vi "GetCaseTerm.vi"(8 "error in (no error)":errorcluster, 9 "CaseStructureName":string, 10 "WireLabel":string, 11 "VI Ref":refnum<vi>) -> (0 "error out":errorcluster, 1 "Open Refs":refnum<vi>[](array[refnum]), 2 "Found?":bool, 3 "Terminal Ref":refnum<vi>)   [LabVIEW 2016, in "CS++Actor.lvlib" / "CS++Actor.lvclass"]
uses:
  CS++Actor.lvclass
  <vilib>/Utility/traverseref.llb/TRef TravTarget.ctl
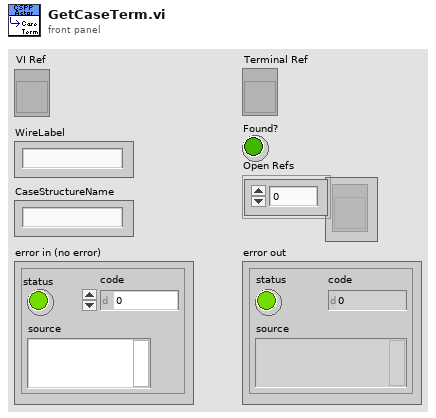
[diagram p1: front panel]
types:
  T1 = typedef "TRef TravTarget.ctl" = enum16{"FP", "BD", "Other"}
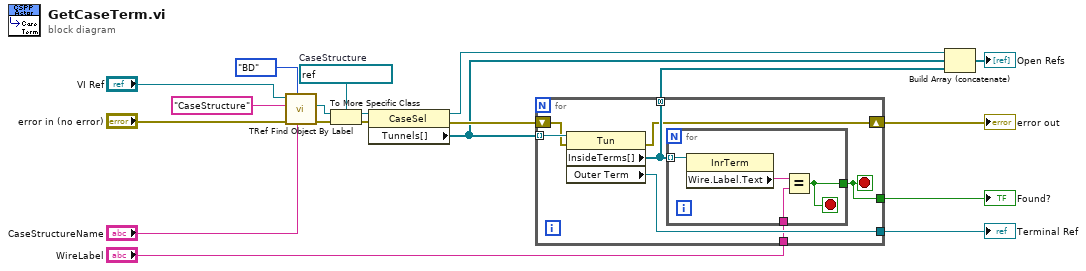
[diagram p0: block diagram]
diagram:
  w17 = refnum<vi> refnum  # CaseStructure
  n1 = call <vilib>:"TRef Find Object By Label.vi"("Label"="CaseStructureName", "Traverse Target"=TRef_TravTarget."BD", "error in (no error)"="error in (no error)", "Class Name"="CaseStructure", "VI Ref"="VI Ref") -> ("error out"=w15:errorcluster, "Found Obj Ref"=w16:refnum<vi>)  [unwired: 3 in, 2 out]
  n2 = To More Specific Class(target class=w17, reference=w16, error in=w15) -> (specific class reference=w18:refnum<vi>, error out=w19:errorcluster)
  n3 = property class="CaseSel"(reference=w18, error in=w19) -> (reference out=w12:refnum<vi>, error out=w11:errorcluster, "Tunnels[]"=w10:refnum<vi>[])
  n4 = for {
    tunnel: w10 -> [w26] mode=indexing
    tunnel: [w25] -> w4
    shift-right: [w20] -> w5
    shift-left: w11 -> [w24]
    tunnel: [w23] -> w9 mode=concatenating
    tunnel: "WireLabel" -> [w22]
    tunnel: [w21] -> w3
    stop <- w21 stop-if-true
    n5 = property class="Tun"(reference=w26, error in=w24) -> (error out=w20:errorcluster, "InsideTerms[]"=w23:refnum<vi>[], "Outer Term"=w25:refnum<vi>)  [unwired: 1 out]
    n6 = for {
      tunnel: w23 -> [w30] mode=indexing
      tunnel: [w28] -> w21
      tunnel: w22 -> [w27]
      stop <- w28 stop-if-true
      n7 = property class="InrTerm"(reference=w30) -> ("Wire.Label.Text"=w29:string)  [unwired: 1 in, 2 out]
      n8 = Equal?(x=w29, y=w27) -> (x = y?=w28:bool)
    }
  }
  "error out" <- w5
  "Terminal Ref" <- w4
  "Found?" <- w3
  n9 = Build Array (concatenate)(w12, w10, w9) -> (→"Open Refs":refnum<vi>[])
